vi "Load VI Into Memory.vi"(8 "error in (no error)":errorcluster, 10 "VI Path":path, 11 "Session in":refnum<class "Session.lvclass">) -> (0 "error out":errorcluster, 3 "Session out":refnum<class "Session.lvclass">)   [LabVIEW 2020, in "Save for Previous Version.lvlib" / "Session.lvclass"]
uses:
  Session.lvclass
  Session.lvclass/Session.ctl
  <userlib>/_OpenG.lib/file/file.llb/Append Path to Root if Relative - Scalar__ogtk.vi
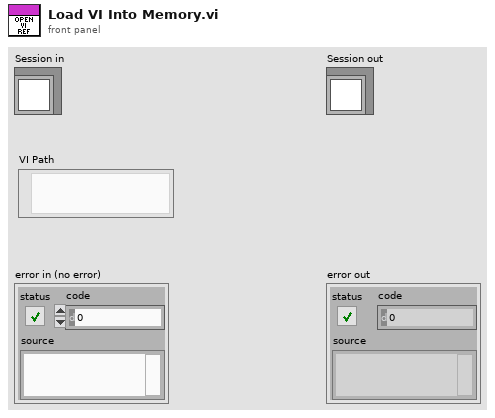
[diagram p1: front panel]
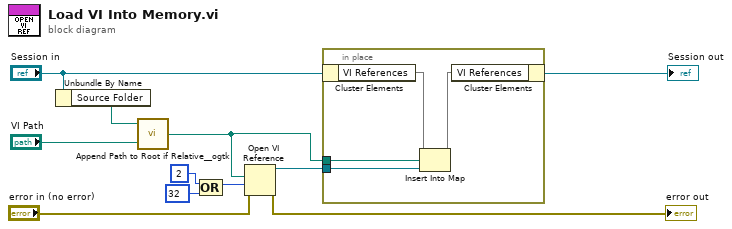
[diagram p0: block diagram]
diagram:
  n1 = Unbundle By Name("Session in") -> ("Source Folder"=w3:path)
  n2 = call-poly <userlib>:"Append Path to Root if Relative__ogtk.vi"("Absolute or Relative Path"="VI Path", "Root Path"=w3) -> ("Absolute or Appended Path"=w1:path)
  n3 = Compound Arithmetic op=OR(2 ("options"), 32 ("options")) -> (w9:i32)
  n4 = Open VI Reference(vi path=w1, options=w9, error in (no error)="error in (no error)") -> (vi reference=w10:refnum<vi>, error out=→"error out":errorcluster)  [unwired: 3 in]
  n5 = in-place {
    in-place-border: w1 -> [w13]
    in-place-border: w10 -> [w12]
    n6 = in-place-cluster #1("Session in") -> ("VI References"=w15:map{path, refnum<vi>})
    n7 = Insert Into Map(map in=w15, key=w13, value=w12) -> (map out=w14:map{path, refnum<vi>})  [unwired: 2 out]
    n8 = in-place-cluster #1("VI References"=w14) -> (→"Session out":refnum<class "Session.lvclass">)
  }
